vi "ChordToAngle.vi"(7 "dL":dbl, 8 "p2Y轴弦长":dbl, 9 "p2X轴弦长":dbl, 10 "p1Y轴弦长":dbl, 11 "p1X轴弦长":dbl) -> (1 "y轴发散角":dbl, 2 "x轴发散角":dbl)   [LabVIEW 2018]
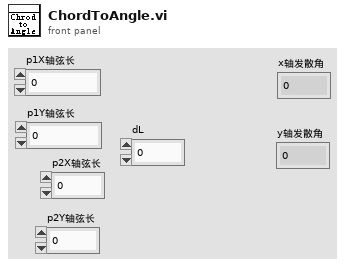
[diagram p1: front panel]
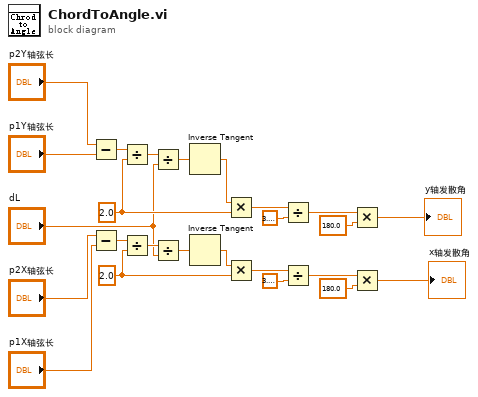
[diagram p0: block diagram]
diagram:
  w12 = 2.0 ("y")
  w21 = 2.0 ("y")
  n1 = Subtract(x="p2Y轴弦长", y="p1Y轴弦长") -> (x-y=w16:dbl)
  n2 = Subtract(x="p2X轴弦长", y="p1X轴弦长") -> (x-y=w25:dbl)
  n3 = Divide(x=w16, y=w12) -> (x/y=w15:dbl)
  n4 = Divide(x=w25, y=w21) -> (x/y=w24:dbl)
  n5 = Divide(x=w15, y="dL") -> (x/y=w14:dbl)
  n6 = Divide(x=w24, y="dL") -> (x/y=w23:dbl)
  n7 = Inverse Tangent(1:w14) -> (0:w13:dbl)
  n8 = Inverse Tangent(1:w23) -> (0:w22:dbl)
  n9 = Multiply(x=w13, y=w12) -> (x*y=w11:dbl)
  n10 = Multiply(x=w22, y=w21) -> (x*y=w20:dbl)
  n11 = Divide(x=w11, y=3.141592653589793) -> (x/y=w9:dbl)
  n12 = Divide(x=w20, y=3.141592653589793) -> (x/y=w18:dbl)
  n13 = Multiply(x=w9, y=180.0) -> (x*y=→"y轴发散角":dbl)
  n14 = Multiply(x=w18, y=180.0) -> (x*y=→"x轴发散角":dbl)
